vi "Read Test Events.vi"(11 "Basic Test Manager in":refnum<class "Basic Test Manager.lvclass">) -> (2 "Test Events":T1, 3 "Basic Test Manager out":refnum<class "Basic Test Manager.lvclass">)   [LabVIEW 2013, in "Caraya.lvlib" / "Basic Test Manager.lvclass"]
uses:
  Basic Test Manager.lvclass
  Test Result/Test Events -- cluster.ctl
  Basic Test Manager.lvclass/Basic Test Manager.ctl
  Test Result/Test Result.lvclass
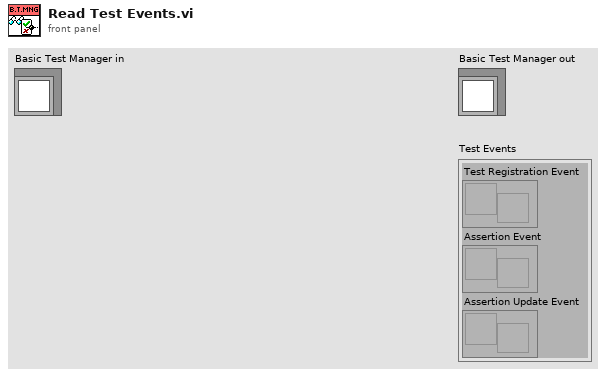
[diagram p1: front panel]
types:
  T1 = typedef "Caraya.lvlib/Test Result.lvclass/Test Events -- cluster.ctl" = cluster{"Test Registration Event":refnum<user-event>, "Assertion Event":refnum<user-event>, "Assertion Update Event":refnum<user-event>}
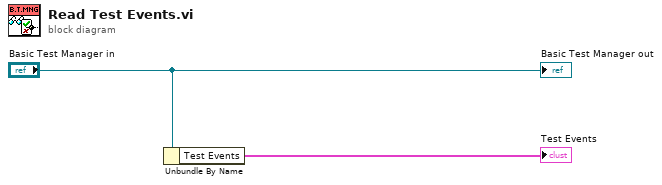
[diagram p0: block diagram]
diagram:
  n1 = Unbundle By Name("Basic Test Manager in") -> ("Test Events"=→"Test Events":T1)
  "Basic Test Manager out" <- "Basic Test Manager in"
